vi "ParseAllClasses.vi"(8 "error in (no error)":errorcluster, 10 "baseClass":refnum<class "baseClass.lvclass">, 11 "baseParser in":refnum<class "baseParser.lvclass">) -> (0 "error out":errorcluster, 2 "AllClasses":refnum<class "baseClass.lvclass">[](array[class]), 3 "baseParser out":refnum<class "baseParser.lvclass">)   [LabVIEW 2013, in "baseParser.lvclass"]
uses:
  baseParser.lvclass
  baseClass/baseClass.lvclass
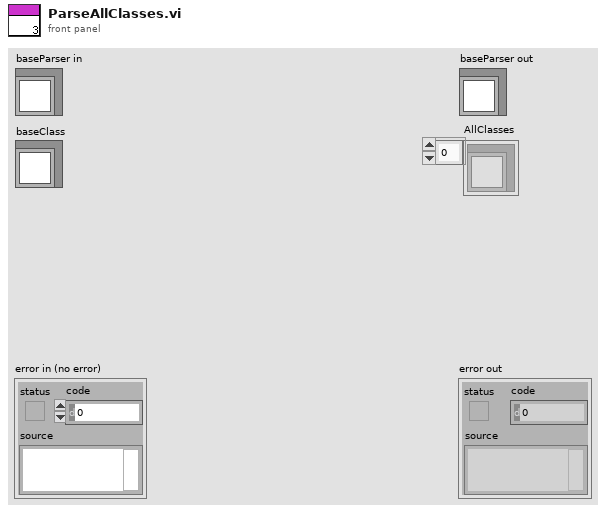
[diagram p1: front panel]
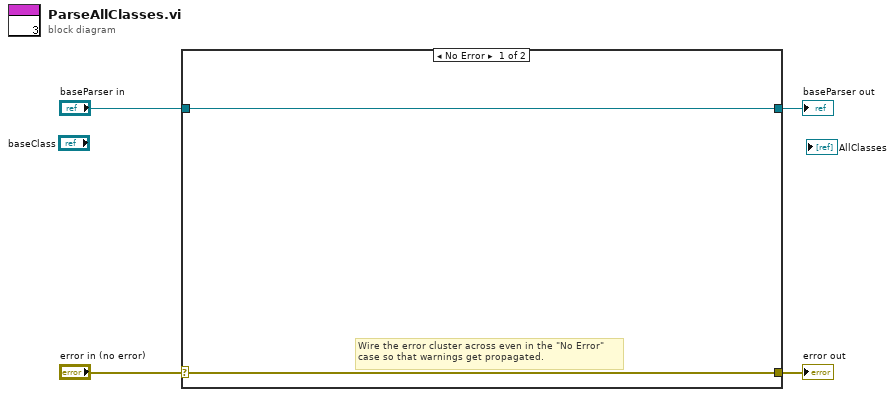
[diagram p0: block diagram]
diagram:
  n1 = case shown="No Error" "error in (no error)" {
    selector: "error in (no error)" -> [w5 w8]
    tunnel: [w5 w8] -> w3
    tunnel: [w6 w7] -> w1
    tunnel: "baseParser in" -> [w6 w7]
    frame No Error {
      # "Wire the error cluster across even in the \"No Error\"\ncase so that warnings get propagated."
    }
    frame Error {
    }
  }
  "error out" <- w3
  "baseParser out" <- w1
